vi "CalcTemp.vi"(8 "error in (no error)":errorcluster, 10 "Adc_temp":i32, 11 "BME68x in":refnum<class "BME680.lvclass">) -> (0 "error out":errorcluster, 2 "Temp":i16, 3 "BME68x out":refnum<class "BME680.lvclass">)   [LabVIEW 2022 SP3, in "BME680.lvlib" / "BME680.lvclass"]
uses:
  BME680.lvclass
  BME680.lvclass/BME680.ctl
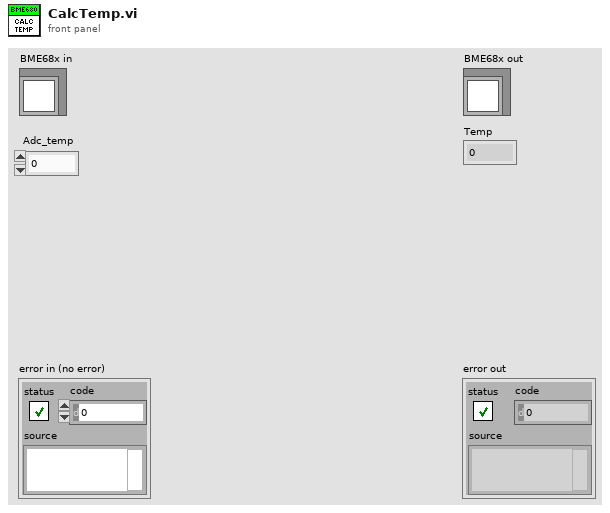
[diagram p1: front panel]
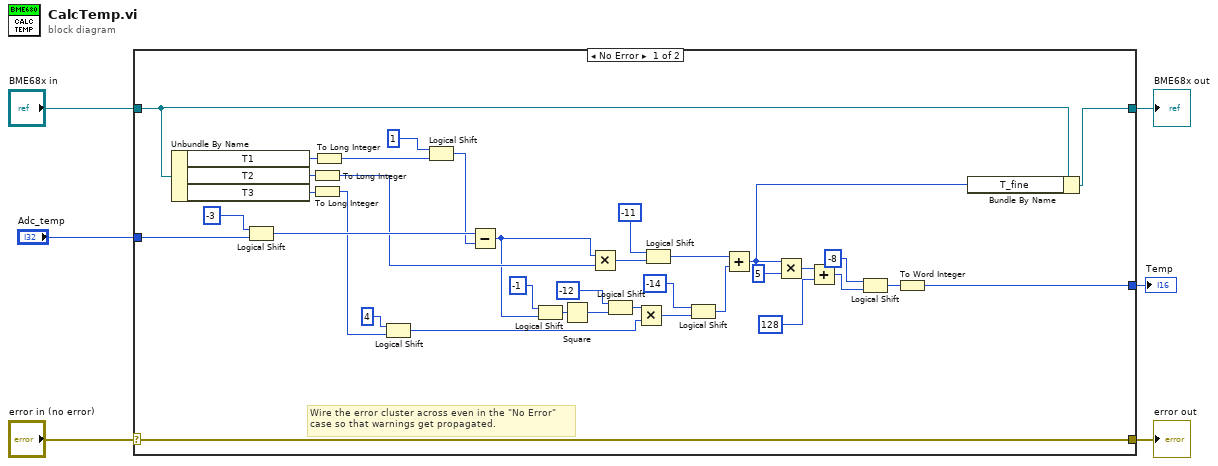
[diagram p0: block diagram]
diagram:
  n1 = case shown="No Error" "error in (no error)" {
    selector: "error in (no error)" -> [w42 w44]
    tunnel: [w42 w44] -> w5
    tunnel: [w40 w43] -> w3
    tunnel: "BME68x in" -> [w41 w43]
    tunnel: "Adc_temp" -> [w21 _]
    tunnel: [w7 _] -> w1
    frame No Error {
      # "Wire the error cluster across even in the \"No Error\"\ncase so that warnings get propagated."
      n2 = Unbundle By Name(w41) -> ("T1"=w39:u16, "T2"=w37:u16, "T3"=w38:u8)
      n3 = Logical Shift(y=-3, x=w21) -> (x << y=w36:i32)
      n4 = To Long Integer(number=w37) -> (32bit integer=w34:i32)
      n5 = To Long Integer(number=w38) -> (32bit integer=w19:i32)
      n6 = To Long Integer(number=w39) -> (32bit integer=w23:i32)
      n7 = Logical Shift(y=4, x=w19) -> (x << y=w31:i32)
      n8 = Logical Shift(y=1, x=w23) -> (x << y=w35:i32)
      n9 = Subtract(x=w36, y=w35) -> (x-y=w17:i32)
      n10 = Logical Shift(y=-1, x=w17) -> (x << y=w33:i32)
      n11 = Square(x=w33) -> (x^2=w11:i32)
      n12 = Multiply(x=w17, y=w34) -> (x*y=w14:i32)
      n13 = Logical Shift(y=-12, x=w11) -> (x << y=w32:i32)
      n14 = Multiply(x=w32, y=w31) -> (x*y=w13:i32)
      n15 = Logical Shift(y=-11, x=w14) -> (x << y=w29:i32)
      n16 = Logical Shift(y=-14, x=w13) -> (x << y=w30:i32)
      n17 = Add(x=w29, y=w30) -> (x+y=w28:i32)
      n18 = Multiply(x=w28, y=5) -> (x*y=w26:i32)
      n19 = Add(x=w26, y=128) -> (x+y=w9:i32)
      n20 = Logical Shift(y=-8, x=w9) -> (x << y=w24:i32)
      n21 = To Word Integer(number=w24) -> (16bit integer=w7:i16)
      n22 = Bundle By Name(cluster=w41, "T_fine"=w28) -> (w40:refnum<class "BME680.lvclass">)
    }
    frame Error {
    }
  }
  "error out" <- w5
  "BME68x out" <- w3
  "Temp" <- w1
